vi "S7COMM - Evaluate Sequence Number.vi"(8 "error in (no error)":errorcluster, 10 "PLC Response Seq No":u16 format="0x%04x", 11 "Sent Seq No.":u16 format="0x%04x") -> (0 "error out":errorcluster)   [LabVIEW 2014, in "S7NetCom.lvclass"]
uses:
  S7NetCom.lvclass
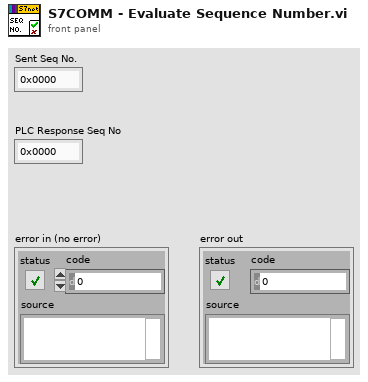
[diagram p1: front panel]
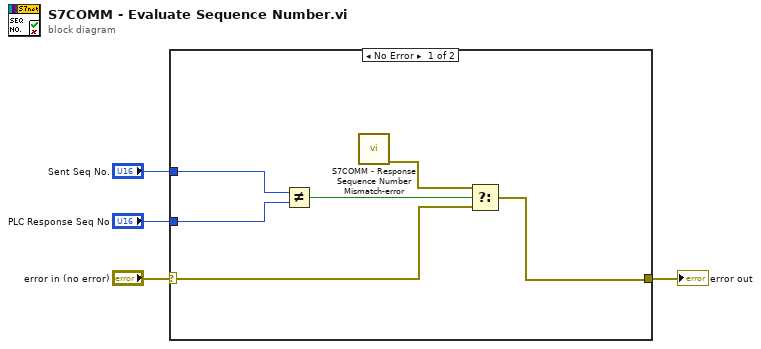
[diagram p0: block diagram]
diagram:
  n1 = case shown="No Error" "error in (no error)" {
    selector: "error in (no error)" -> [w7 w11]
    tunnel: [w6 w11] -> w4
    tunnel: "Sent Seq No." -> [w10 _]
    tunnel: "PLC Response Seq No" -> [w9 _]
    frame No Error {
      n2 = Not Equal?(x=w10, y=w9) -> (x != y?=w8:bool)
      n3 = call "S7COMM - Response Sequence Number Mismatch-error.vi"() -> ("error out"=w5:errorcluster)  [unwired: 11 in]
      n4 = Select(t=w5, s=w8, f=w7) -> (s? t:f=w6:errorcluster)
    }
    frame Error {
    }
  }
  "error out" <- w4
